vi "NISE.Read Register (Core).vi"(0 "SLSC Interface in":refnum<class "SLSC Interface.lvclass">, 1 "type":enum16{"U8", "U16", "U32", "U64"}(ring), 5 "device":refnum<k21>="$DefaultDevices", 7 "register address":u32 format="%.0x", 11 "error in (no error)":errorcluster) -> (4 "SLSC Interface out":refnum<class "SLSC Interface.lvclass">, 6 "device out":refnum<k21>, 8 "next register address":u32 format="%.0x", 10 "data out":u64 format="%.0x", 15 "error out":errorcluster)   [LabVIEW 2016, in "SLSC Interface.lvclass"]
uses:
  SLSC Interface.lvclass
  SLSC Interface.lvclass/SLSC Interface.ctl
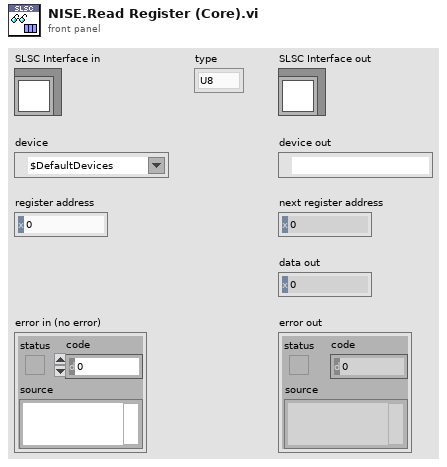
[diagram p1: front panel]
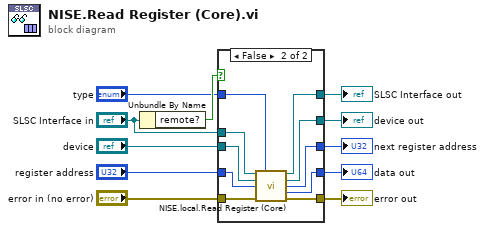
[diagram p0: block diagram]
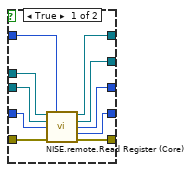
[diagram p2: hidden frame]
diagram:
  n1 = Unbundle By Name("SLSC Interface in") -> ("remote?"=w11:bool)
  n2 = case shown="False" w11 {
    tunnel: "SLSC Interface in" -> [w21 w31]
    tunnel: "type" -> [w20 w30]
    tunnel: [w19 w29] -> w9
    tunnel: "device" -> [w18 w28]
    tunnel: [w17 w27] -> w7
    tunnel: "register address" -> [w16 w26]
    tunnel: [w15 w25] -> w5
    tunnel: [w14 w24] -> w4
    tunnel: "error in (no error)" -> [w13 w23]
    tunnel: [w12 w22] -> w2
    frame True {
      n3 = call "NISE.remote.Read Register (Core).vi"("SLSC Remote in"=w21, "type"=w20, "device"=w18, "register address"=w16, "error in (no error)"=w13) -> ("SLSC Remote out"=w19:refnum<class "SLSC Interface.lvclass">, "device out"=w17:refnum<k21>, "next register address"=w15:u32, "data out"=w14:u64, "error out"=w12:errorcluster)  [unwired: 6 in]
    }
    frame False {
      n4 = call "NISE.local.Read Register (Core).vi"("SLSC Local in"=w31, "type"=w30, "device"=w28, "register address"=w26, "error in (no error)"=w23) -> ("SLSC Local out"=w29:refnum<class "SLSC Interface.lvclass">, "device out"=w27:refnum<k21>, "next register address"=w25:u32, "data out"=w24:u64, "error out"=w22:errorcluster)  [unwired: 6 in]
    }
  }
  "error out" <- w2
  "SLSC Interface out" <- w9
  "device out" <- w7
  "next register address" <- w5
  "data out" <- w4
